vi "OnDataChange.vi"(0 "TripleAxisStageController in":refnum<class "TriaxesStageController.lvclass">, 1 "DataExchange":T1, 3 "error in (no error)":errorcluster) -> (7 "TripleAxisStageController out":refnum<class "TriaxesStageController.lvclass">, 10 "error out":errorcluster)   [LabVIEW 2020, in "TriaxesStageController.lvlib" / "TriaxesStageController.lvclass"]
uses:
  TriaxesStageController.lvclass
  Model/Hardware Abstraction Layer/Component/Device/Device/DataExchange.ctl
  Interface/DataListener/DataListener.lvclass
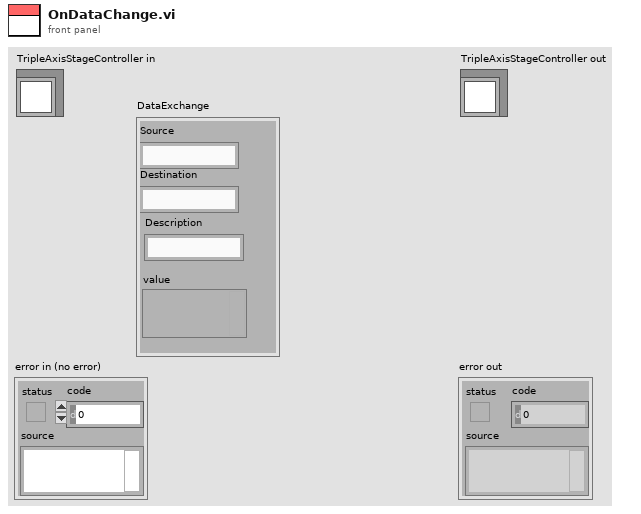
[diagram p1: front panel]
types:
  T1 = typedef "DataListener.lvclass/DataExchange.ctl" = cluster{"Source":string, "Destination":string, "Description":string, "value":variant}
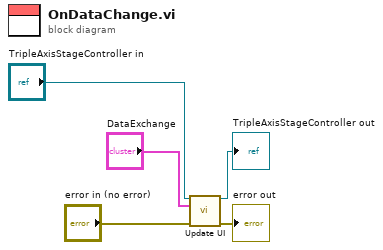
[diagram p0: block diagram]
diagram:
  n1 = call-dynamic "Update UI.vi"("Stage Controller in"="TripleAxisStageController in", "DataExchange"="DataExchange", "error in (no error)"="error in (no error)") -> ("Stage Controller out"=→"TripleAxisStageController out":refnum<class "TriaxesStageController.lvclass">, "error out"=→"error out":errorcluster)  [unwired: 11 in]
